vi "xy_init.vi"(9 "y number":dbl, 10 "x number":dbl) -> (3 "xy":dbl[][](array[numeric]))   [LabVIEW 2013]
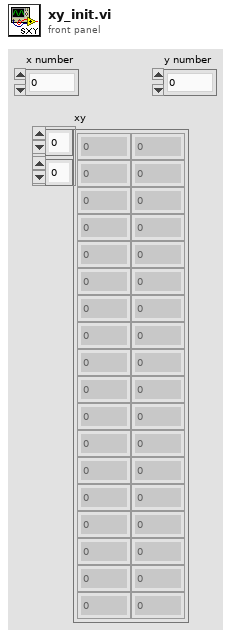
[diagram p1: front panel]
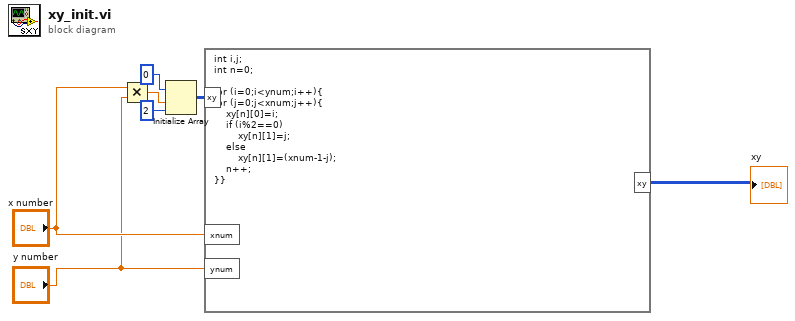
[diagram p0: block diagram]
diagram:
  n1 = Multiply(x="x number", y="y number") -> (x*y=w5:dbl)
  n2 = Initialize Array(0, w5, 2) -> (w3:i32[][])
  n3 = formula code="int i,j;\nint n=0;\n\nfor (i=0;i<ynum;i++){\nfor (j=0;j<xnum;j++){\n    xy[n][0]=i;\n    if (i%2==0)\n        xy[n][1]=j;\n    else\n        xy[n][1]=(xnum-1-j);\n    n++;\n}}"("xnum"="x number", "ynum"="y number", "xy"=w3) -> ("xy"=→"xy":i32[][])
